vi "setTwoToneSignal.vi"(7 "Channel":string="0", 8 "error in (no error)":errorcluster, 9 "tone amplitudes":dbl format="%.2p", 10 "tone frequencies":dbl format="%.2p", 11 "Fgen.lvclass":refnum<class "Arb.lvclass">) -> (0 "error out":errorcluster, 3 "Fgen.lvclass out":refnum<class "Arb.lvclass">)   [LabVIEW 2023, in "sweArb.lvlib" / "Arb.lvclass"]
doc: "<b>Author:</b> Wolfgang\n<b>Description:</b> Apply a two tone signal"
uses:
  Arb.lvclass
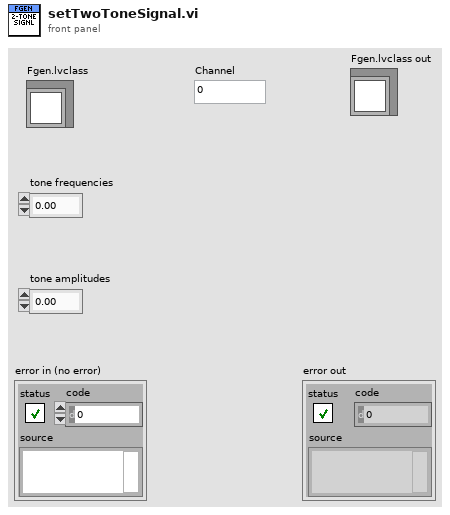
[diagram p1: front panel]
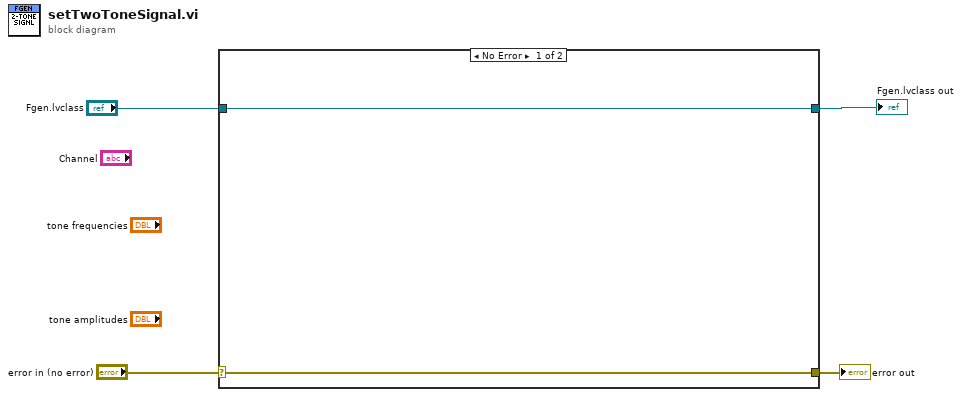
[diagram p0: block diagram]
diagram:
  n1 = case shown="No Error" "error in (no error)" {
    selector: "error in (no error)" -> [w5 w8]
    tunnel: [w5 w8] -> w3
    tunnel: [w6 w7] -> w1
    tunnel: "Fgen.lvclass" -> [w6 w7]
    frame No Error {
    }
    frame Error {
    }
  }
  "error out" <- w3
  "Fgen.lvclass out" <- w1
